vi "st_eval CDF (chisq).vi"(4 "parameters":variant, 5 "x":dbl) -> (2 "f(x)":dbl)   [LabVIEW 2017, in "NI_Gmath.lvlib"]
uses:
  <vilib>/gmath/NI_Gmath.lvlib
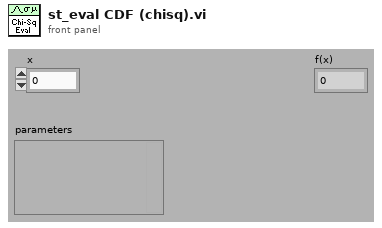
[diagram p1: front panel]
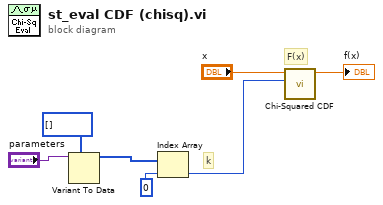
[diagram p0: block diagram]
diagram:
  # "k"
  # "F(x)"
  n1 = Variant To Data(type=i32[] [], Variant="parameters") -> (data=w5:i32[])  [unwired: 1 in, 1 out]
  n2 = Index Array(array=w5, index=0) -> (element=w1:i32)
  n3 = call <vilib>:"Chi-Squared CDF.vi"("k"=w1, "x"="x") -> ("cdf(x)"=→"f(x)":dbl)  [unwired: 8 in, 1 out]
